vi "ex7-14.vi"() -> ()   [LabVIEW 2013]
panel:
  out "appended array":dbl[][](array[numeric])
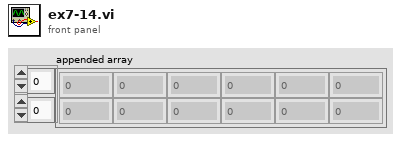
[diagram p1: front panel]
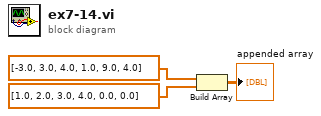
[diagram p0: block diagram]
diagram:
  n1 = Build Array(dbl[] [-3.0, 3.0, 4.0, 1.0, 9.0, 4.0] ("array"), dbl[] [1.0, 2.0, 3.0, 4.0, 0.0, 0.0] ("array")) -> (→"appended array":dbl[][])
